vi "collectLT_img.vi"() -> (0 "cts/sec":dbl, 1 "counts":i32)   [LabVIEW 2013]
uses:
  phlib.dll
panel:
  out "buffer size":i32
  out "time elapsed":u32
  out "iterations":i32=5
  out "counts per\niteration":i32[](array[numeric])
  out "trunc buffer":u32[](array[numeric]) format="%08x"
  out "buffer":u32[](array[numeric]) format="%08x"
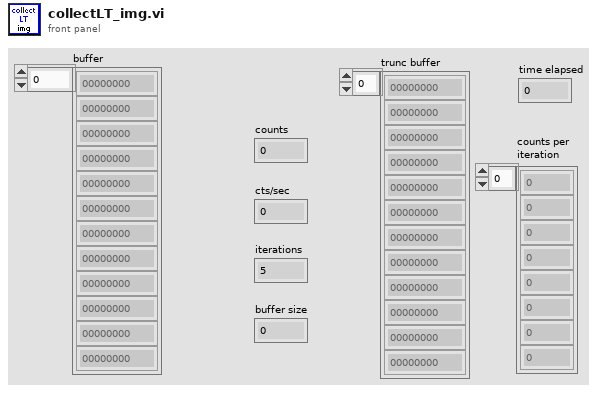
[diagram p1: front panel]
types:
  T1 = cluster{"Z_n":i32[], "initialized":bool, "devidx":i32, "Ch0 Level":i32, "Ch0 ZeroX":i32, "Ch1 Level":i32, "Ch1 ZeroX":i32, "sync rate":i32, "resolution":i32, "acq time":i32, "acq rate":i32, "# bins":u32, "Bin size":enum16{"1", "2", "4", "8", "16", "32", "64", "128"}, "min photons":u32, "truncate":u32}
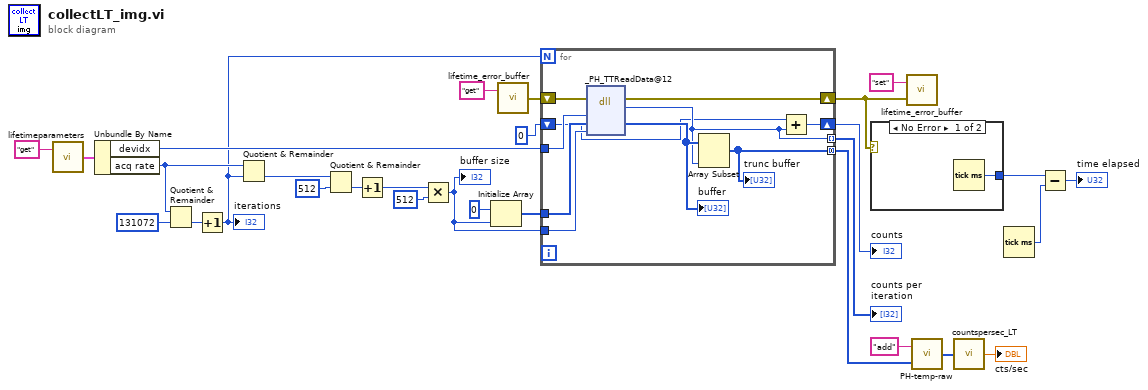
[diagram p0: block diagram]
diagram:
  n1 = call "lifetimeparameters.vi"("command"="get") -> ("Params out"=w24:T1)  [unwired: 1 in]
  n2 = Unbundle By Name(w24) -> ("devidx"=w23:i32, "acq rate"=w9:i32)
  n3 = Quotient & Remainder(x=w9, y=131072) -> (floor(x/y)=w8:i32)  [unwired: 1 out]
  n4 = Increment(x=w8) -> (x+1=w7:i32)
  "iterations" <- w7
  n5 = Quotient & Remainder(x=w9, y=w7) -> (floor(x/y)=w3:i32)  [unwired: 1 out]
  n6 = Quotient & Remainder(x=w3, y=512) -> (floor(x/y)=w4:i32)  [unwired: 1 out]
  n7 = Increment(x=w4) -> (x+1=w6:i32)
  n8 = Multiply(x=w6, y=512) -> (x*y=w5:i32)
  "buffer size" <- w5
  n9 = Initialize Array(u32 0, w5) -> (w16:u32[])
  n10 = call "lifetime_error_buffer.vi"("command"="get") -> ("error out"=w26:errorcluster)  [unwired: 1 in]
  n11 = for {
    N: w7 -> [_]
    tunnel: w23 -> [w36]
    shift-right: [w37] -> w11
    shift-left: w26 -> [w38]
    tunnel: [w32] -> w21 mode=indexing
    tunnel: [w35] -> w19 mode=concatenating
    tunnel: w16 -> [w34]
    tunnel: w5 -> [w33]
    shift-right: [w31] -> w15
    shift-left: 0 ("return type") -> [w30]
    n12 = dll-call lib="phlib.dll" fn="_PH_TTReadData@12" label="PH_TTReadData"(error in=w38, "devidx"=w36, "buffer"=w34, "blocksize"=w33) -> (error out=w37:errorcluster, "return type"=w32:i32, "buffer"=w39:u32[])  [unwired: 4 in, 1 out]
    "buffer" <- w39
    n13 = Array Subset(array=w39, length=w32) -> (w35:u32[])  [unwired: 1 in]
    "trunc buffer" <- w35
    n14 = Add(x=w30, y=w32) -> (x+y=w31:i32)
  }
  "counts per\niteration" <- w21
  "counts" <- w15
  n15 = case shown="No Error" w11 {
    tunnel: [w40 _] -> w13
    frame No Error {
      n16 = Tick Count (ms)() -> (millisecond timer value=w40:u32)
    }
    frame Error {
    }
  }
  n17 = call "lifetime_error_buffer.vi"("error in"=w11, "command"="set") -> ()  [unwired: 1 out]
  n18 = call "PH-temp-raw.vi"("array in"=w19, "command"="add") -> ("array out"=w18:u32[])
  n19 = call "countspersec_LT.vi"("1D PH data"=w18) -> ("Avg cts/s"=→"cts/sec":dbl)
  n20 = Tick Count (ms)() -> (millisecond timer value=w29:u32)
  n21 = Subtract(x=w13, y=w29) -> (x-y=→"time elapsed":u32)
